vi "P9MagnetMonitor.vi"() -> ()   [LabVIEW 2019]
uses:
  Utility/Monitor Communication/PPMS/P9_P14_Magnet-cluster.ctl
  Global/Global Variables/Data_Display_global.vi
  Instrument_Setup.vi
panel:
  in  "stop":bool
  out "error out":errorcluster
  in  "error in (no error)":errorcluster
  in  "P9/P14-Magnet-Cluster":T1 {"Magnet Status" items=["MagnetUnknown"=0, "StablePersistent"=1, "WarmingSwitch"=2, "CoolingSwitch"=3, "StableDriven"=4, "Iterating"=5, "Charging"=6, "Discharging"=7, "CurrentError"=8, "MagnetFailure"=15]; "Approach" items=["Linear", "NoOvershoot", "Oscillate"]}
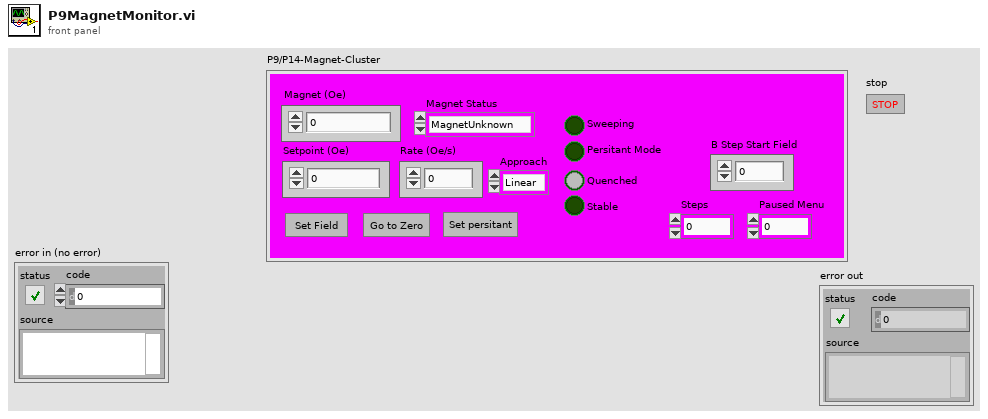
[diagram p1: front panel]
types:
  T1 = typedef "P9_P14_Magnet-cluster.ctl" = cluster{"Magnet (Oe)":dbl, "Setpoint (Oe)":dbl, "Rate (Oe/min)":dbl, "Set Field":bool, "Go to zero":bool, "Set Persitant/non-pers":bool, "Approach":i32, "Magnet Status":i32, "Sweeping":bool, "Quenched":bool, "Persitant Mode ":bool, "Stable":bool, "Steps":dbl, "Paused Menu":dbl, "B Step Start Field":dbl}
  T2 = typedef "P9P14_Magnet_Control.ctl" = cluster{"Setpoint (Oe)":dbl, "Rate (Oe/min)":dbl, "Set Field":bool, "Go to zero":bool, "Set Persitant/non-pers":bool, "Approach":i32, "Steps":dbl, "Paused Menu":dbl, "B Step start Field":dbl}
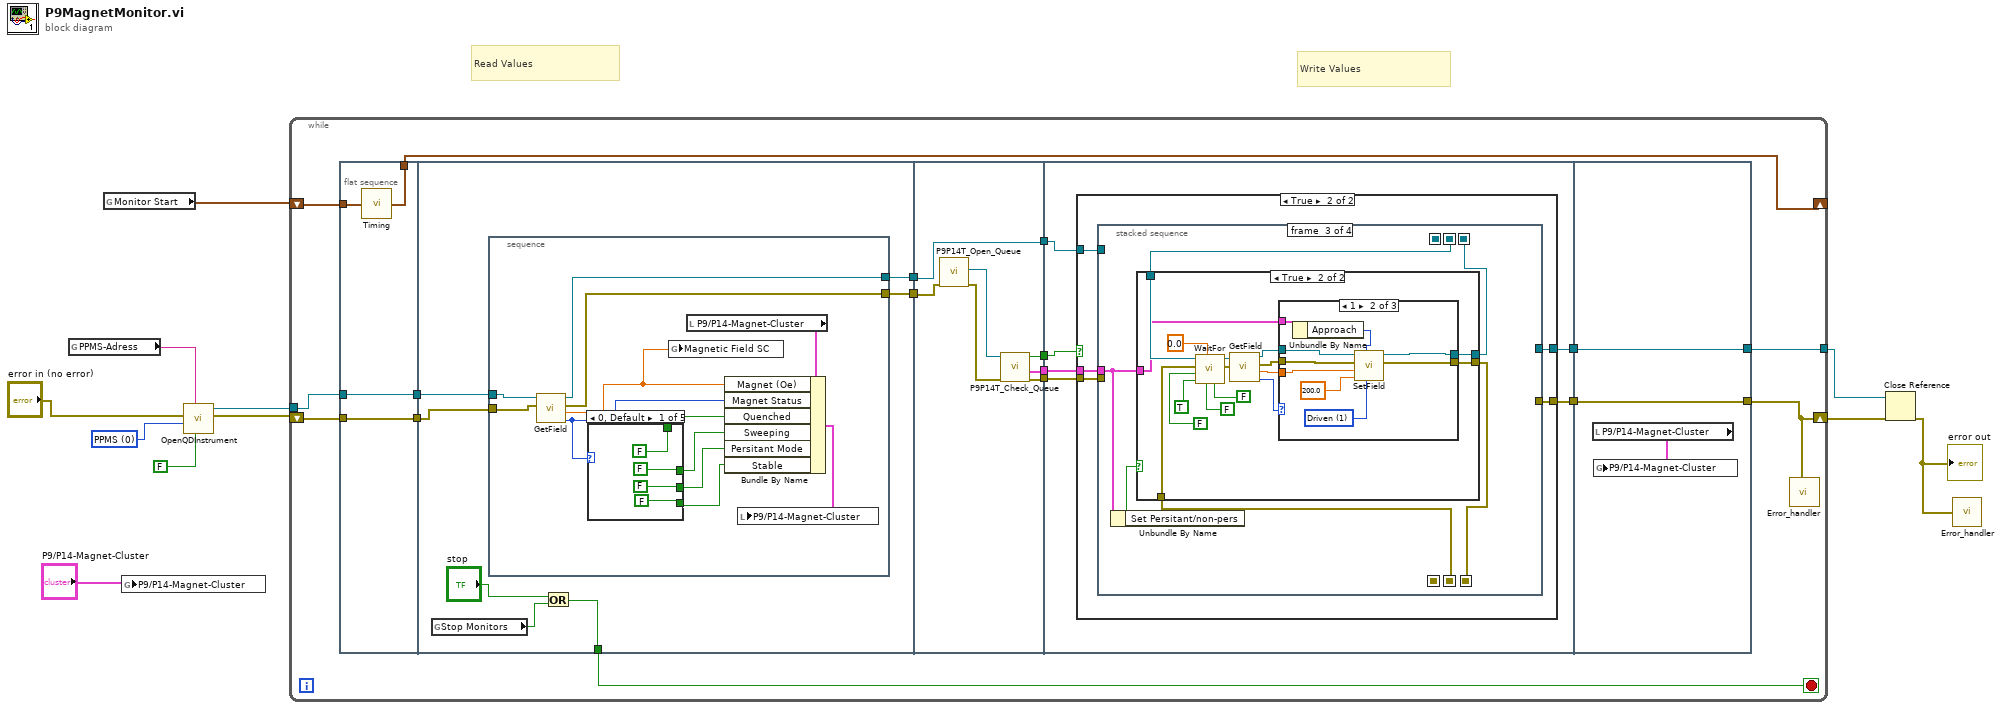
[diagram p0: block diagram]
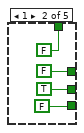
[diagram p2: hidden frame]
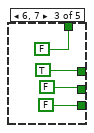
[diagram p3: hidden frame]
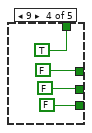
[diagram p4: hidden frame]
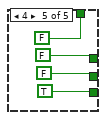
[diagram p5: hidden frame]
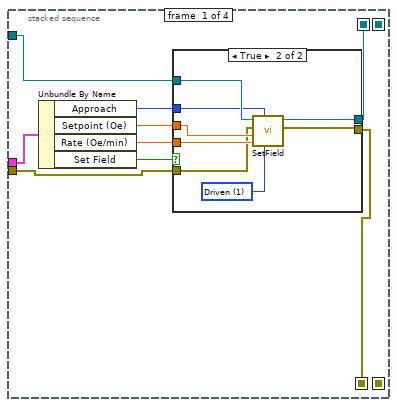
[diagram p7: hidden frame]
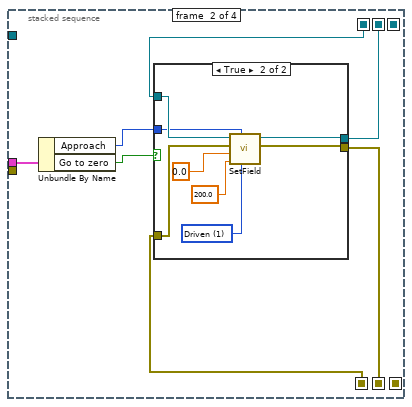
[diagram p9: hidden frame]
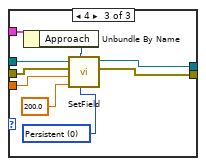
[diagram p13: hidden frame]
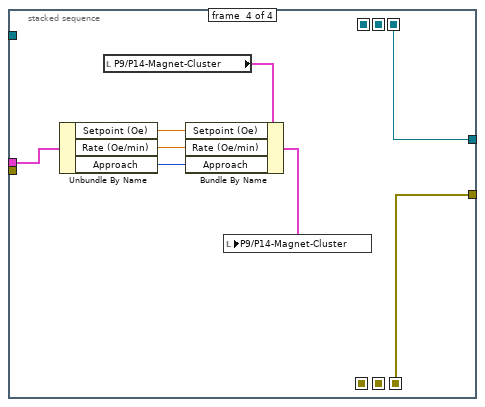
[diagram p14: hidden frame]
diagram:
  w9 = 0 items=["PPMS", "VersaLab", "DynaCool", "SVSM", "OptiCool"] ("InstrumentType")
  # "Write Values"
  # "Read Values"
  n1 = global read "Instrument_Setup.vi" "PPMS-Adress"() -> (w8:string)
  n2 = global read "Data_Display_global.vi" "Monitor Start"() -> (w11:timestamp)
  n3 = global write "Data_Display_global.vi" "P9/P14-Magnet-Cluster"("P9/P14-Magnet-Cluster") -> ()
  n4 = call "OpenQDInstrument.vi"("Remote"=FALSE, "IP Address"=w8, "InstrumentType"=w9, "error in (no error)"="error in (no error)") -> ("error out"=w10:errorcluster, "Instrument Ref"=w6:refnum<k24>)  [unwired: 4 in]
  n5 = while {
    shift-right: [w24] -> _
    shift-left: w11 -> [w28]
    shift-right: [w12] -> w2
    shift-left: w10 -> [w26]
    tunnel: w6 -> [w22]
    tunnel: [w13] -> w1
    stop <- w27 stop-if-true
    n6 = flat-sequence {
      tunnel: w26 -> [w31]
      tunnel: w28 -> [w32]
      tunnel: [w31] -> w25
      tunnel: [w30] -> w24
      tunnel: [w29] -> w23
      tunnel: w22 -> [w29]
      tunnel: [w37] -> w27
      tunnel: w25 -> [w36]
      tunnel: w23 -> [w35]
      tunnel: [w34] -> w21
      tunnel: [w33] -> w20
      tunnel: w21 -> [w72]
      tunnel: w20 -> [w78]
      tunnel: [w75] -> w19
      tunnel: [w74] -> w18
      tunnel: [w73] -> w17
      tunnel: [w72] -> w16
      tunnel: w19 -> [w84]
      tunnel: w18 -> [w83]
      tunnel: w17 -> [w82]
      tunnel: w16 -> [w81]
      tunnel: [w80] -> w15
      tunnel: [w79] -> w14
      tunnel: w15 -> [w180]
      tunnel: w14 -> [w181]
      tunnel: [w181] -> w13
      tunnel: [w180] -> w12
      frame #0 {
        n7 = call "Timing.vi"("start time (s)"=w32) -> ("last reading (s)"=w30:timestamp)
      }
      frame #1 {
        n8 = global read "Data_Display_global.vi" "Stop Monitors"() -> (w38:bool)
        n9 = stacked-sequence {
          tunnel: w36 -> [w51]
          tunnel: w35 -> [w50]
          tunnel: [w46] -> w34
          tunnel: [w45] -> w33
          frame #0 {
            n10 = call "GetField.vi"("error in (no error)"=w51, "Instrument Ref In"=w50) -> ("Field\nStatus"=w47:i32, "Field"=w41:dbl, "error out"=w45:errorcluster, "Instrument Ref Out"=w46:refnum<k24>)  [unwired: 3 in, 1 out]
            n11 = case shown="0, Default" w47 {
              tunnel: [FALSE FALSE FALSE TRUE FALSE] -> w44
              tunnel: [FALSE FALSE TRUE FALSE FALSE] -> w43
              tunnel: [FALSE TRUE FALSE FALSE FALSE] -> w42
              tunnel: [FALSE FALSE FALSE FALSE TRUE] -> w40
              frame 0, Default {
              }
              frame 1 {
              }
              frame 6, 7 {
              }
              frame 9 {
              }
              frame 4 {
              }
            }
            n12 = global write "Data_Display_global.vi" "Magnetic Field SC"(w41) -> ()
            n13 = local read "P9/P14-Magnet-Cluster"() -> (w49:T1)
            n14 = Bundle By Name(cluster=w49, "Magnet (Oe)"=w41, "Magnet Status"=w47, "Quenched"=w44, "Sweeping"=w43, "Persitant Mode"=w42, "Stable"=w40) -> (w48:T1)
            n15 = local write "P9/P14-Magnet-Cluster"(w48) -> ()
          }
        }
        n16 = Or(x="stop", y=w38) -> (x .or. y?=w37:bool)
      }
      frame #2 {
        n17 = call "P9P14T_Open_Queue.vi"("error in (no error)"=w78) -> ("error out"=w77:errorcluster, "queue out"=w76:refnum<queue>)  [unwired: 9 in]
        n18 = call "P9P14T_Check_Queue.vi"("error in (no error)"=w77, "queue"=w76) -> ("error out"=w73:errorcluster, "P9/P14-Magnet-Control"=w74:T2, "New Entries?"=w75:bool)  [unwired: 6 in]
      }
      frame #3 {
        n19 = case shown="True" w84 {
          tunnel: w83 -> [_ w91]
          tunnel: w82 -> [w85 w90]
          tunnel: w81 -> [w86 w89]
          tunnel: [w86 w88] -> w79
          tunnel: [w85 w87] -> w80
          frame False {
          }
          frame True {
            n20 = stacked-sequence {
              seq-local: [w94 _ _ _] -> [_ w115 _ _]
              seq-local: [w93 _ _ _] -> [_ w114 _ _]
              seq-local: [_ w112 _ _] -> [_ _ w131 _]
              seq-local: [_ w111 _ _] -> [_ _ w130 _]
              seq-local: [_ _ w129 _] -> [_ _ _ w173]
              seq-local: [_ _ w128 _] -> [_ _ _ w172]
              tunnel: w91 -> [w100 w117 w132 w179]
              tunnel: w90 -> [w95 _ _ _]
              tunnel: w89 -> [w96 _ _ _]
              tunnel: [_ _ _ w173] -> w88
              tunnel: [_ _ _ w172] -> w87
              frame #0 {
                n21 = Unbundle By Name(w100) -> ("Approach"=w92:i32, "Setpoint (Oe)"=w98:dbl, "Rate (Oe/min)"=w97:dbl, "Set Field"=w99:bool)
                n22 = case shown="True" w99 {
                  tunnel: w98 -> [_ w110]
                  tunnel: w97 -> [_ w109]
                  tunnel: w96 -> [w102 w108]
                  tunnel: w95 -> [w101 w107]
                  tunnel: [w102 w105] -> w94
                  tunnel: [w101 w104] -> w93
                  tunnel: w92 -> [_ w103]
                  frame False {
                  }
                  frame True {
                    w106 = 1 items=["Persistent", "Driven"] ("Mode")
                    n23 = call "SetField.vi"("Mode"=w106, "Approach"=w103, "Rate"=w109, "Field"=w110, "error in (no error)"=w107, "Instrument Ref In"=w108) -> ("error out"=w104:errorcluster, "Instrument Ref Out"=w105:refnum<k24>)  [unwired: 1 in, 1 out]
                  }
                }
              }
              frame #1 {
                n24 = Unbundle By Name(w117) -> ("Approach"=w113:i32, "Go to zero"=w116:bool)
                n25 = case shown="True" w116 {
                  tunnel: w115 -> [w119 w127]
                  tunnel: w114 -> [w118 w126]
                  tunnel: [w119 w124] -> w112
                  tunnel: [w118 w121] -> w111
                  tunnel: w113 -> [_ w120]
                  frame False {
                  }
                  frame True {
                    w122 = 1 items=["Persistent", "Driven"] ("Mode")
                    n26 = call "SetField.vi"("Mode"=w122, "Approach"=w120, "Rate"=200.0, "Field"=0.0, "error in (no error)"=w126, "Instrument Ref In"=w127) -> ("error out"=w121:errorcluster, "Instrument Ref Out"=w124:refnum<k24>)  [unwired: 1 in, 1 out]
                  }
                }
              }
              frame #2 {
                n27 = Unbundle By Name(w132) -> ("Set Persitant/non-pers"=w133:bool)
                n28 = case shown="True" w133 {
                  tunnel: w132 -> [_ w138]
                  tunnel: w131 -> [w135 w144]
                  tunnel: w130 -> [w134 w143]
                  tunnel: [w135 w137] -> w129
                  tunnel: [w134 w136] -> w128
                  frame False {
                  }
                  frame True {
                    n29 = call "WaitFor.vi"("Wait For Chamber"=FALSE, "Wait For Position"=FALSE, "Delay"=0.0, "Wait For Field"=TRUE, "Wait For Temperature"=FALSE, "error in (no error)"=w143, "Instrument Ref In"=w144) -> ("error out"=w145:errorcluster, "Instrument Ref Out"=w146:refnum<k24>)  [unwired: 3 in]
                    n30 = call "GetField.vi"("error in (no error)"=w145, "Instrument Ref In"=w146) -> ("Field\nStatus"=w151:i32, "Field"=w148:dbl, "error out"=w149:errorcluster, "Instrument Ref Out"=w150:refnum<k24>)  [unwired: 3 in, 1 out]
                    n31 = case shown="1" w151 {
                      tunnel: w150 -> [w153 w162 w171]
                      tunnel: w149 -> [w152 w161 w170]
                      tunnel: w148 -> [_ w160 w169]
                      tunnel: w138 -> [_ w158 w166]
                      tunnel: [w153 w155 w164] -> w137
                      tunnel: [w152 w154 w163] -> w136
                      frame 0, Default {
                      }
                      frame 1 {
                        w156 = 1 items=["Persistent", "Driven"] ("Mode")
                        n32 = Unbundle By Name(w158) -> ("Approach"=w157:i32)
                        n33 = call "SetField.vi"("Mode"=w156, "Approach"=w157, "Rate"=200.0, "Field"=w160, "error in (no error)"=w161, "Instrument Ref In"=w162) -> ("error out"=w154:errorcluster, "Instrument Ref Out"=w155:refnum<k24>)  [unwired: 1 in, 1 out]
                      }
                      frame 4 {
                        w167 = 0 items=["Persistent", "Driven"] ("Mode")
                        n34 = Unbundle By Name(w166) -> ("Approach"=w165:i32)
                        n35 = call "SetField.vi"("Mode"=w167, "Approach"=w165, "Rate"=200.0, "Field"=w169, "error in (no error)"=w170, "Instrument Ref In"=w171) -> ("error out"=w163:errorcluster, "Instrument Ref Out"=w164:refnum<k24>)  [unwired: 1 in, 1 out]
                      }
                    }
                  }
                }
              }
              frame #3 {
                n36 = Unbundle By Name(w179) -> ("Setpoint (Oe)"=w177:dbl, "Rate (Oe/min)"=w176:dbl, "Approach"=w175:i32)
                n37 = local read "P9/P14-Magnet-Cluster"() -> (w178:T1)
                n38 = Bundle By Name(cluster=w178, "Setpoint (Oe)"=w177, "Rate (Oe/min)"=w176, "Approach"=w175) -> (w174:T1)
                n39 = local write "P9/P14-Magnet-Cluster"(w174) -> ()
              }
            }
          }
        }
      }
      frame #4 {
        n40 = local read "P9/P14-Magnet-Cluster"() -> (w182:T1)
        n41 = global write "Data_Display_global.vi" "P9/P14-Magnet-Cluster"(w182) -> ()
      }
    }
    n42 = call "Error_handler.vi"("error constant"=w12) -> ()
  }
  n43 = Close Reference(reference=w1, error in (no error)=w2) -> (error out=w4:errorcluster)
  "error out" <- w4
  n44 = call "Error_handler.vi"("error constant"=w4) -> ()
